vi "SAOMM-DataFlow.vi"() -> ()   [LabVIEW 2011]
panel:
  out "Centroids":cluster{dbl[], dbl[]}[](graph)
  out "Flux":cluster{dbl[], dbl[]}[](graph)
  in  "pattern":string="*"
  out "SNR":cluster{dbl[], dbl[]}[](graph)
  out "subimg":u8[][](graph)
  in  "Target ExecTime":u32=25
  in  "DataLenght":dbl
  out "HexpodXGraph":cluster{dbl[], dbl[]}[](graph)
  out "Filename":path
  in  "DirPath":path=path "C:/BonOMM/BonOMM-2012/Syslogs/Hexapod/CommandLoggingClosedLoop"
  out "Cumulatif":cluster{dbl[], dbl[]}[](graph)
  out "ExecTime":u32=45
  out "ErrorYGraph":cluster{dbl[], dbl[]}[](graph)
  in  "Quit":bool
  # "FalconProcessed"
  # "CommandLogging"
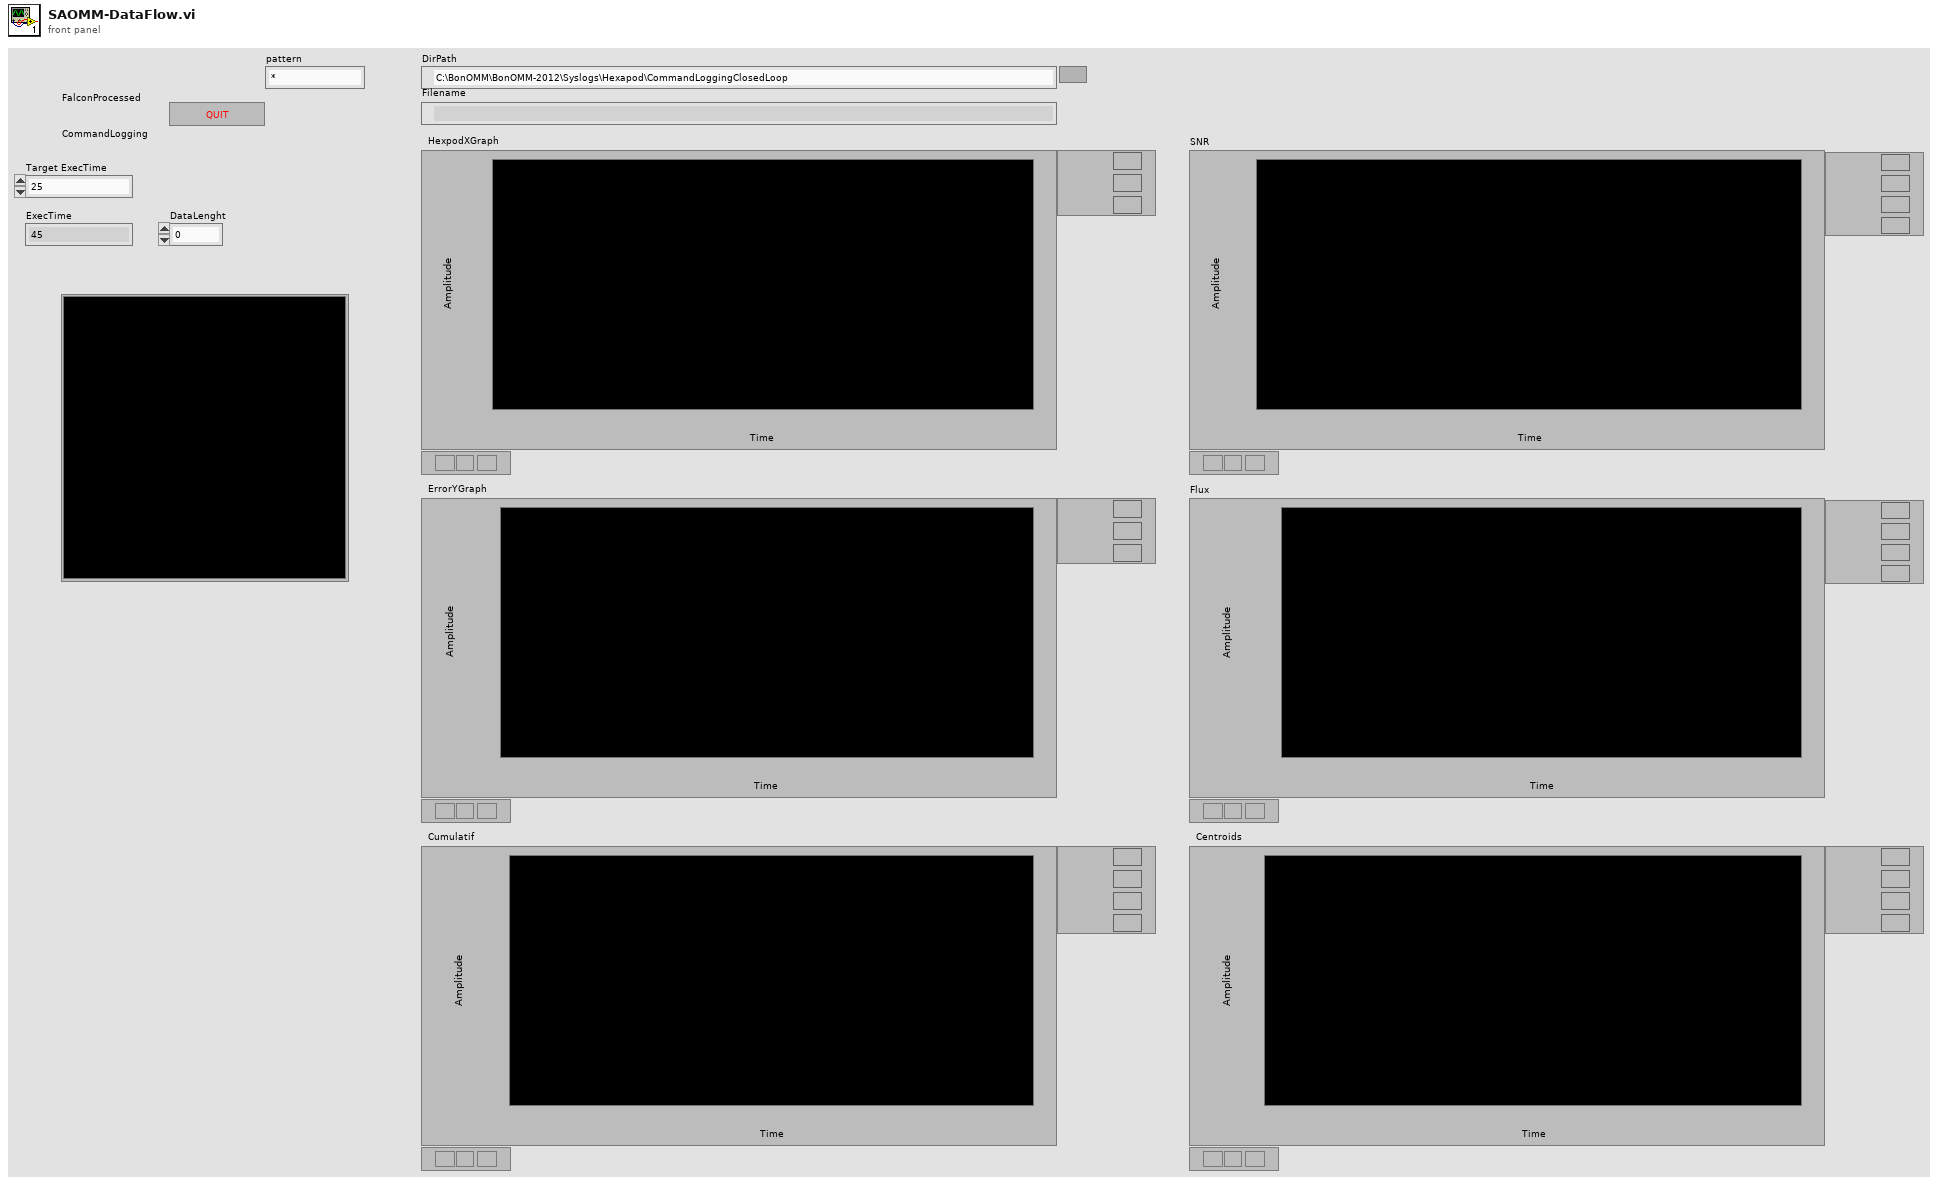
[diagram p1: front panel]
types:
  T1 = cluster{"Logging ID":u32, "Logging TimeStapmp":u64, "Azimuth":dbl, "Elevation":dbl, "Rotation":dbl, "ServoLevel":u16, "ROIWidth":u16, "ROIHeight":u16, "ROIXOffset":u16, "ROIYOffset":u16, "Pixel X":dbl, "Pixel Y":dbl, "ImageTimeStamp":u64, "CommandTimeStamp":u64, "Flux":dbl, "SNR":dbl, "SNRTreshold":dbl, "CentroidX":dbl, "CentroidY":dbl}
  T2 = cluster{"Hexapod_Nominal":dbl[], "Hexapod_Offset":dbl[], "Hexapod_LUT":dbl[], "Hexapod_ServoX":dbl[], "Hexapode_ServoY":dbl[], "Hexapod_Console":dbl[], "Hexapod_Position":dbl[], "Hexapod_Command":dbl[], "Hexapod_Filtered":dbl[]}
  T3 = cluster{"SNR":dbl, "SNRTreshold":dbl, "Flux":dbl}
  T4 = cluster{"ROIXOffset":u16, "CentroidX":dbl, "Pixel X":dbl, "ROIYOffset":u16, "CentroidY":dbl, "Pixel Y":dbl}
  T5 = cluster{"Largeur de l'image":dbl, "Hauteur de l'image":dbl, "Bits par Pixel":dbl, "ID de l'image":u32, "Frame Rate":dbl, "Largeur de Bande":dbl, "Time Stamp":u64}
  T6 = cluster{"Largeur de la ROI":u16, "Hauteur de la ROI":u16, "Position X de la ROI":u16, "Position Y de la ROI":u16, "Minimum de la ROI":u32, "Maximum de la ROI":u32}
  T7 = cluster{"Seuil du masque":dbl, "Flux":dbl, "SNR":dbl, "Centroide X":dbl, "Centroide Y":dbl}
  T8 = cluster{"Position X de la ROI":u16, "Centroide X":dbl, dbl, "Position Y de la ROI":u16, "Centroide Y":dbl, dbl}
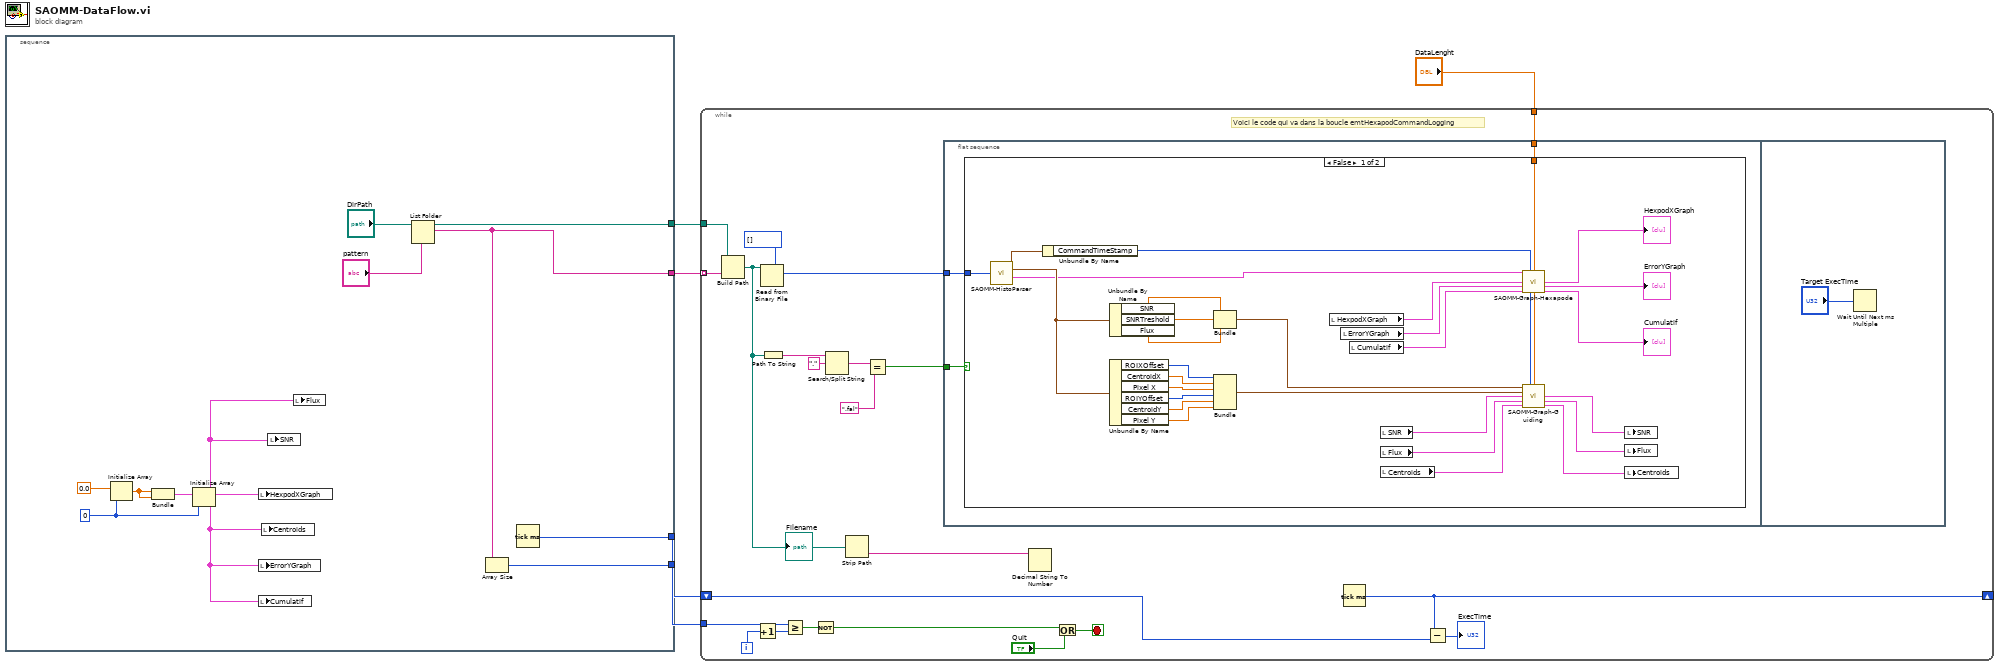
[diagram p0: block diagram]
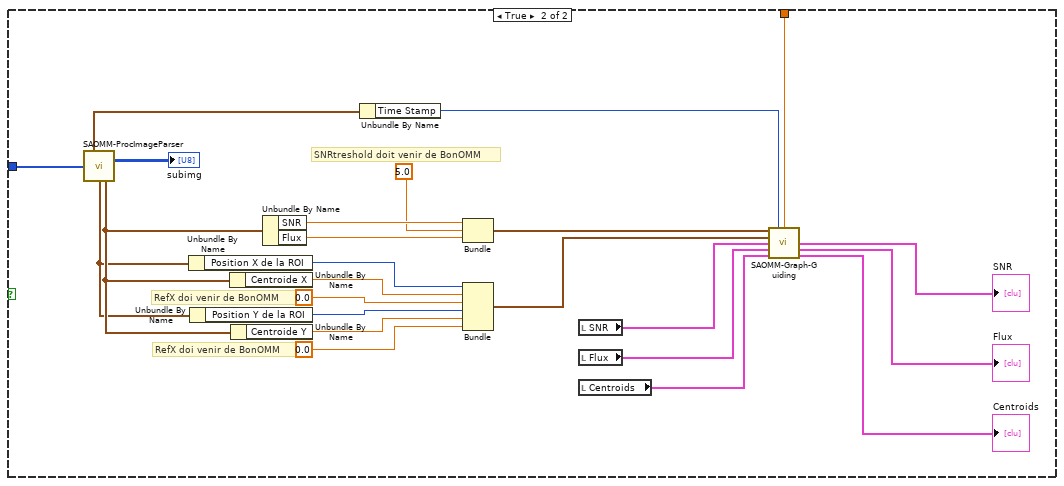
[diagram p2: hidden frame]
diagram:
  n1 = stacked-sequence {
    tunnel: [w16] -> w5
    tunnel: [w15] -> w4
    tunnel: [w9] -> w3
    tunnel: [w10] -> w1
    frame #0 {
      w7 = 0 ("millisecond multiple")
      n2 = Initialize Array(0.0, w7) -> (w13:dbl[])
      n3 = Bundle(w13, w13) -> (w8:cluster{dbl[], dbl[]})  [unwired: 1 in]
      n4 = Initialize Array(w8, w7) -> (w6:cluster{dbl[], dbl[]}[])
      n5 = local write "HexpodXGraph"(w6) -> ()
      n6 = local write "ErrorYGraph"(w6) -> ()
      n7 = local write "Cumulatif"(w6) -> ()
      n8 = local write "Centroids"(w6) -> ()
      n9 = local write "SNR"(w6) -> ()
      n10 = local write "Flux"(w6) -> ()
      n11 = List Folder(path="DirPath", pattern="pattern") -> (path out=w10:path, filenames=w9:string[])  [unwired: 2 in, 2 out]
      n12 = Array Size(array=w9) -> (size(s)=w16:i32)
      n13 = Tick Count (ms)() -> (millisecond timer value=w15:u32)
    }
  }
  n14 = while {
    tunnel: w3 -> [w28] mode=indexing
    tunnel: w5 -> [w35]
    shift-right: [w30] -> _
    shift-left: w4 -> [w31]
    tunnel: "DataLenght" -> [w26]
    tunnel: w1 -> [w24]
    i -> [w34]
    stop <- w36 stop-if-true
    # "Voici le code qui va dans la boucle emtHexapodCommandLogging"
    n15 = Build Path(base path=w24, name or relative path=w28) -> (appended path=w18:path)
    "Filename" <- w18
    n16 = Increment(x=w34) -> (x+1=w27:i32)
    n17 = Read from Binary File(5:u8[] [], 11:w18) -> (2:w25:u8[])  [unwired: 4 in, 3 out]
    n18 = Path To String(path=w18) -> (string=w19:string)
    n19 = Greater Or Equal?(x=w35, y=w27) -> (x >= y?=w33:bool)
    n20 = Not(x=w33) -> (.not. x?=w32:bool)
    n21 = Search/Split String(string=w19, search string/char (-)=".") -> (match + rest of string=w20:string)  [unwired: 1 in, 2 out]
    n22 = Strip Path(path=w18) -> (name=w17:string)  [unwired: 1 out]
    n23 = Equal?(x=w20, y=".fal") -> (x = y?=w22:bool)
    n24 = flat-sequence {
      tunnel: w26 -> [w41]
      tunnel: w25 -> [w40]
      tunnel: w22 -> [w39]
      frame #0 {
        n25 = case shown="False" w39 {
          tunnel: w41 -> [w59 w91]
          tunnel: w40 -> [w69 w93]
          frame False {
            n26 = call "SAOMM-HistoParser.vi"("DataStream"=w69) -> ("Source cluster"=w50:T1, "Hexapod cluster"=w42:T2)  [unwired: 13 in]
            n27 = Unbundle By Name(w50) -> ("CommandTimeStamp"=w55:u64)
            n28 = Unbundle By Name(w50) -> ("SNR"=w53:dbl, "SNRTreshold"=w54:dbl, "Flux"=w52:dbl)
            n29 = Unbundle By Name(w50) -> ("ROIXOffset"=w49:u16, "CentroidX"=w48:dbl, "Pixel X"=w47:dbl, "ROIYOffset"=w46:u16, "CentroidY"=w45:dbl, "Pixel Y"=w44:dbl)
            n30 = Bundle("SNR"=w53, "SNRTreshold"=w54, "Flux"=w52) -> (w51:T3)  [unwired: 1 in]
            n31 = Bundle("ROIXOffset"=w49, "CentroidX"=w48, "Pixel X"=w47, "ROIYOffset"=w46, "CentroidY"=w45, "Pixel Y"=w44) -> (w43:T4)  [unwired: 1 in]
            n32 = local read "HexpodXGraph"() -> (w67:cluster{dbl[], dbl[]}[])
            n33 = local read "ErrorYGraph"() -> (w68:cluster{dbl[], dbl[]}[])
            n34 = local read "Cumulatif"() -> (w64:cluster{dbl[], dbl[]}[])
            n35 = local read "SNR"() -> (w62:cluster{dbl[], dbl[]}[])
            n36 = local read "Flux"() -> (w61:cluster{dbl[], dbl[]}[])
            n37 = local read "Centroids"() -> (w60:cluster{dbl[], dbl[]}[])
            n38 = call "SAOMM-Graph-Hexapode.vi"("Hexapod cluster"=w42, "LoggingTimeStamp"=w55, "DataLenght (seconds)"=w59, "X IN"=w67, "Y IN"=w68, "Cumul IN"=w64) -> ("X OUT"=→"HexpodXGraph":cluster{dbl[], dbl[]}[], "Y OUT"=→"ErrorYGraph":cluster{dbl[], dbl[]}[], "Cumul OUT"=→"Cumulatif":cluster{dbl[], dbl[]}[])  [unwired: 7 in]
            n39 = call "SAOMM-Graph-Guiding.vi"("SNR Data"=w51, "TimeStamp"=w55, "DataLenght (seconds)"=w59, "Centroids Data"=w43, "SNR IN"=w62, "Flux IN"=w61, "Centroids IN"=w60) -> ("SNR OUT"=w58:cluster{dbl[], dbl[]}[], "Flux OUT"=w57:cluster{dbl[], dbl[]}[], "Centroids OUT"=w56:cluster{dbl[], dbl[]}[])  [unwired: 6 in]
            n40 = local write "SNR"(w58) -> ()
            n41 = local write "Flux"(w57) -> ()
            n42 = local write "Centroids"(w56) -> ()
          }
          frame True {
            # "RefX doi venir de BonOMM"
            # "RefX doi venir de BonOMM"
            # "SNRtreshold doit venir de BonOMM"
            n43 = call "SAOMM-ProcImageParser.vi"("ProcessedData"=w93) -> ("GrayLevels"=→"subimg":u8[][], "GeneralProperties"=w71:T5, "ROIProperties"=w79:T6, "ProcessedProperties"=w80:T7)  [unwired: 8 in, 3 out]
            n44 = Unbundle By Name(w79) -> ("Position X de la ROI"=w74:u16)
            n45 = Unbundle By Name(w79) -> ("Position Y de la ROI"=w77:u16)
            n46 = Unbundle By Name(w80) -> ("Centroide X"=w72:dbl)
            n47 = Unbundle By Name(w80) -> ("Centroide Y"=w75:dbl)
            n48 = Unbundle By Name(w80) -> ("SNR"=w87:dbl, "Flux"=w83:dbl)
            n49 = Unbundle By Name(w71) -> ("Time Stamp"=w70:u64)
            n50 = Bundle("SNR"=w87, 5.0, "Flux"=w83) -> (w81:cluster{"SNR":dbl, dbl, "Flux":dbl})  [unwired: 1 in]
            n51 = Bundle("Position X de la ROI"=w74, "Centroide X"=w72, 0.0, "Position Y de la ROI"=w77, "Centroide Y"=w75, 0.0) -> (w76:T8)  [unwired: 1 in]
            n52 = local read "SNR"() -> (w84:cluster{dbl[], dbl[]}[])
            n53 = local read "Flux"() -> (w85:cluster{dbl[], dbl[]}[])
            n54 = local read "Centroids"() -> (w86:cluster{dbl[], dbl[]}[])
            n55 = call "SAOMM-Graph-Guiding.vi"("SNR Data"=w81, "TimeStamp"=w70, "DataLenght (seconds)"=w91, "Centroids Data"=w76, "SNR IN"=w84, "Flux IN"=w85, "Centroids IN"=w86) -> ("SNR OUT"=→"SNR":cluster{dbl[], dbl[]}[], "Flux OUT"=→"Flux":cluster{dbl[], dbl[]}[], "Centroids OUT"=→"Centroids":cluster{dbl[], dbl[]}[])  [unwired: 6 in]
          }
        }
      }
      frame #1 {
        n56 = Wait Until Next ms Multiple(millisecond multiple="Target ExecTime") -> ()  [unwired: 1 out]
      }
    }
    n57 = Decimal String To Number(string=w17) -> ()  [unwired: 2 in, 2 out]
    n58 = Or(x=w32, y="Quit") -> (x .or. y?=w36:bool)
    n59 = Tick Count (ms)() -> (millisecond timer value=w30:u32)
    n60 = Subtract(x=w30, y=w31) -> (x-y=→"ExecTime":u32)
  }
